vi "Set Default Value.vi"(9 "Default C++ Value":string, 10 "Control Ref":refnum<vi>, 11 "Abstract Param Writer in":refnum<class "Abstract Param Writer.lvclass">) -> (1 "LabVIEW Default String":string, 2 "Control Ref Dup":refnum<vi>, 3 "Abstract Param Writer out":refnum<class "Abstract Param Writer.lvclass">)   [LabVIEW 2013, in "Abstract Param Writer.lvclass"]
doc: "Copyright (c) 2016 Sze Howe Koh\n\nThis Source Code Form is subject to the terms of the Mozilla Public License, v. 2.0. If a copy of the MPL was not distributed with this file, You can obtain one at http://mozilla.org/MPL/2.0/."
uses:
  Abstract Param Writer.lvclass
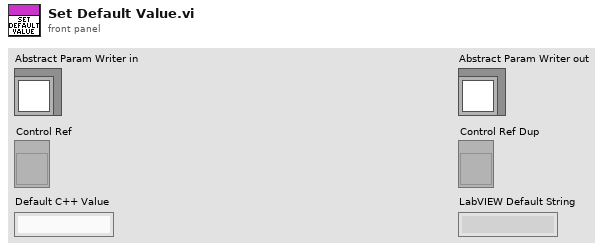
[diagram p1: front panel]
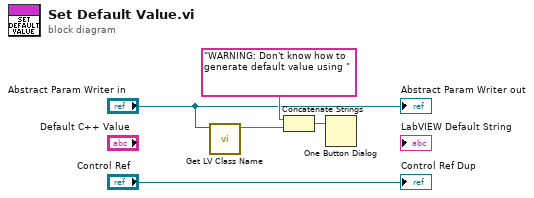
[diagram p0: block diagram]
diagram:
  n1 = call <vilib>:"Get LV Class Name.vi"("object"="Abstract Param Writer in") -> ("class name"=w4:string)  [unwired: 9 in, 1 out]
  n2 = Concatenate Strings("WARNING: Don't know how to generate default value using ", w4) -> (w2:string)
  n3 = One Button Dialog(message=w2) -> ()  [unwired: 1 in, 1 out]
  "Abstract Param Writer out" <- "Abstract Param Writer in"
  "Control Ref Dup" <- "Control Ref"
